vi "general-scan-stopping-criteria.vi"(7 "reset":bool=TRUE, 9 "scan-status":T1={"boolean \nindicators"={"unstable-z-traj"=FALSE, "input fifo time-out"=FALSE, "logging fifo timeout"=FALSE, "scanning finished"=FALSE, "unstable-x-traj"=FALSE, "unstable-y-traj"=FALSE, "ABORT"=FALSE, "All Measurements Done"=FALSE, "fpga_finished"=FALSE, "current_scan_finished"=FALSE}, "current-state"=0, "z-u(k)"=0.0, "number-settled-samples-x"=0, "number-settled-samples-y"=0, "number-settled-samples-Z"=0, "scan-idx"=0, "state-counts"=[0, 0, 0, 0, 0, 0]}, 10 "current-state":u8, 11 "FIFO-elementas-left":u8) -> (3 "Finish":bool)   [LabVIEW 2017]
uses:
  fpga_VIs/controls/fpga-scan-status.ctl
  controls/boolean_info.ctl
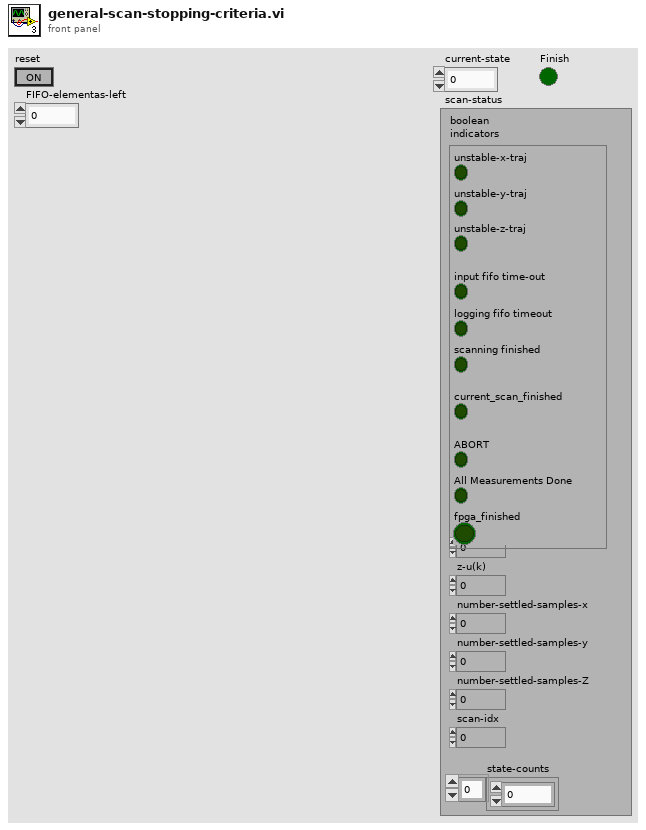
[diagram p1: front panel]
types:
  T1 = typedef "fpga-scan-status.ctl" = cluster{"boolean \nindicators":T2, "current-state":u8, "z-u(k)":sgl, "number-settled-samples-x":i16, "number-settled-samples-y":i16, "number-settled-samples-Z":i16, "scan-idx":i16, "state-counts":u64[]}
  T2 = typedef "boolean_info.ctl" = cluster{"unstable-z-traj":bool, "input fifo time-out":bool, "logging fifo timeout":bool, "scanning finished":bool, "unstable-x-traj":bool, "unstable-y-traj":bool, "ABORT":bool, "All Measurements Done":bool, "fpga_finished":bool, "current_scan_finished":bool}
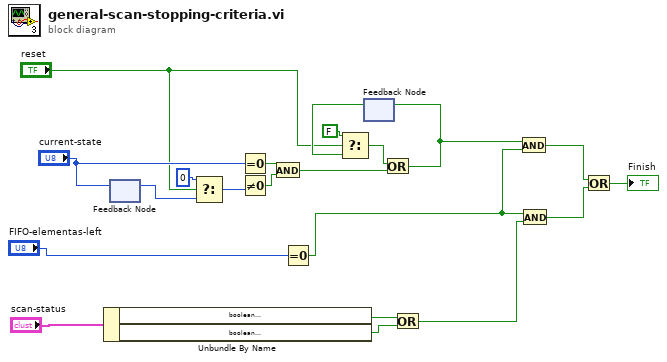
[diagram p0: block diagram]
diagram:
  n1 = Unbundle By Name("scan-status") -> ("boolean \nindicators.unstable-z-traj"=w8:bool, "boolean \nindicators.fpga_finished"=w9:bool)
  n2 = feedback #1() -> (w13:u8)  [unwired: 1 in]
  n3 = feedback-in #1("current-state") -> ()
  n4 = Select(t=u8 0, s="reset", f=w13) -> (s? t:f=w14:u8)
  n5 = Equal To 0?(x="current-state") -> (x = 0?=w21:bool)
  n6 = Not Equal To 0?(x=w14) -> (x != 0?=w20:bool)
  n7 = And(x=w21, y=w20) -> (x .and. y?=w19:bool)
  n8 = Equal To 0?(x="FIFO-elementas-left") -> (x = 0?=w5:bool)
  n9 = feedback #2() -> (w16:bool)  [unwired: 1 in]
  n10 = Select(t=FALSE, s="reset", f=w16) -> (s? t:f=w17:bool)
  n11 = Or(x=w17, y=w19) -> (x .or. y?=w4:bool)
  n12 = feedback-in #2(w4) -> ()
  n13 = Or(x=w8, y=w9) -> (x .or. y?=w6:bool)
  n14 = And(x=w4, y=w5) -> (x .and. y?=w3:bool)
  n15 = And(x=w5, y=w6) -> (x .and. y?=w2:bool)
  n16 = Or(x=w3, y=w2) -> (x .or. y?=→"Finish":bool)
